vi "Configure Valve.vi"(6 "Three Way Valve Position (0:None)":u16(ring) items=["None", "Bypass", "Input", "Output"], 7 "Valve Type (0:None)":u16(ring) items=["None", "3 Way Non-Distribution", "3 Way Distribution", "4 Way Non-Distribution", "4 Way Distribution", "5 Way Non-Distribution", "5 Way Distribution", "6 Way Non-Distribution", "6 Way Distribution", "8 Way Non-Distribution", "8 Way Distribution", "12 Way Distribution", "2 Way Non-Distribution"], 8 "error in (no error)":errorcluster, 9 "Valve Position (1:Port A)":u16(ring)=1 items=["Port A"=1, "Port B"=2, "Port C"=3, "Port D"=4, "Port E"=5, "Port F"=6, "Port G"=7, "Port H"=8, "Port I"=9, "Port J"=10, "Port K"=11, "Port L"=12], 10 "Address (1)":u16=1 max=15 step=1, 11 "VISA resource name":refnum<visa-resource-name>) -> (0 "error out":errorcluster, 3 "VISA resource name out":refnum<visa-resource-name>)   [LabVIEW 2021, in "Copy of Kloehn V6 Series.lvlib"]
doc: "Configures properties of the valve for the instrument. Things that are customizable include valve type and valve position. It is possible to have more than valve which can be connected via the built in ports or the expansion ports. For those valves that are three way, there are some more options for the positioning of the valve."
uses:
  Copy of Kloehn V6 Series.lvlib
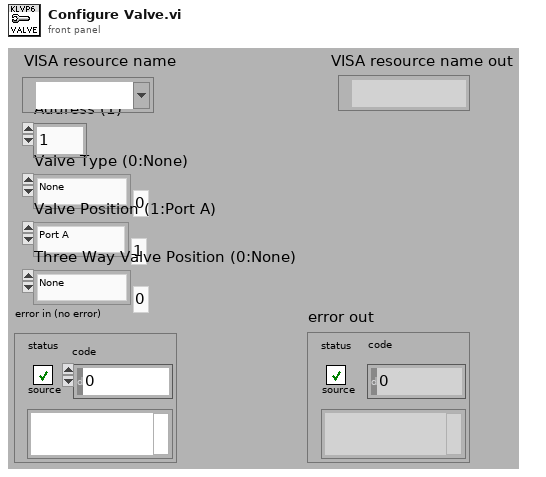
[diagram p1: front panel]
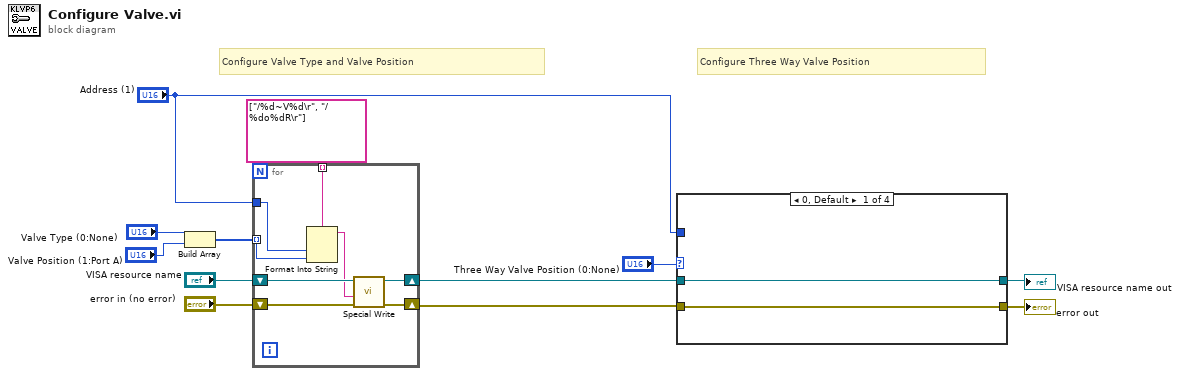
[diagram p0: block diagram]
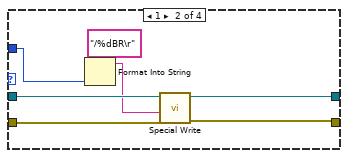
[diagram p2: hidden frame]
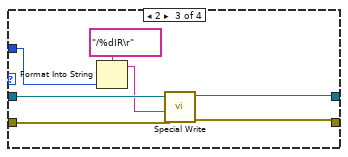
[diagram p3: hidden frame]
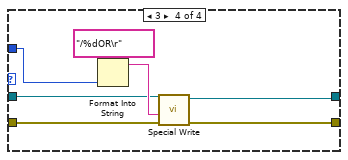
[diagram p4: hidden frame]
diagram:
  # "Configure Three Way Valve Position"
  # "Configure Valve Type and Valve Position"
  n1 = Build Array("Valve Type (0:None)", "Valve Position (1:Port A)") -> (w8:u16[])
  n2 = for {
    tunnel: string[] ["/%d~V%d\r", "/%do%dR\r"] -> [w13] mode=indexing
    tunnel: w8 -> [w20] mode=indexing
    shift-right: [w18] -> w6
    shift-left: "VISA resource name" -> [w17]
    shift-right: [w15] -> w5
    shift-left: "error in (no error)" -> [w14]
    tunnel: "Address (1)" -> [w19]
    n3 = Format Into String(format string=w13, w19, w20) -> (resulting string=w16:string)  [unwired: 2 in, 1 out]
    n4 = call "Special Write.vi"("error in (no error)"=w14, "Send String"=w16, "VISA resource name"=w17) -> ("error out"=w15:errorcluster, "VISA resource name out"=w18:refnum<visa-resource-name>)  [unwired: 4 in, 3 out]
  }
  n5 = case shown="0, Default" "Three Way Valve Position (0:None)" {
    tunnel: [w22 w23 w30 w37] -> w2
    tunnel: w6 -> [w22 w27 w34 w40]
    tunnel: [w21 w24 w31 w38] -> w4
    tunnel: w5 -> [w21 w25 w32 w39]
    tunnel: "Address (1)" -> [_ w29 w35 w42]
    frame 0, Default {
    }
    frame 1 {
      n6 = Format Into String(format string="/%dBR\r" ("Send String"), w29) -> (resulting string=w26:string)  [unwired: 2 in, 1 out]
      n7 = call "Special Write.vi"("error in (no error)"=w25, "Send String"=w26, "VISA resource name"=w27) -> ("error out"=w24:errorcluster, "VISA resource name out"=w23:refnum<visa-resource-name>)  [unwired: 4 in, 3 out]
    }
    frame 2 {
      n8 = Format Into String(format string="/%dIR\r" ("Send String"), w35) -> (resulting string=w33:string)  [unwired: 2 in, 1 out]
      n9 = call "Special Write.vi"("error in (no error)"=w32, "Send String"=w33, "VISA resource name"=w34) -> ("error out"=w31:errorcluster, "VISA resource name out"=w30:refnum<visa-resource-name>)  [unwired: 4 in, 3 out]
    }
    frame 3 {
      n10 = Format Into String(format string="/%dOR\r" ("Send String"), w42) -> (resulting string=w41:string)  [unwired: 2 in, 1 out]
      n11 = call "Special Write.vi"("error in (no error)"=w39, "Send String"=w41, "VISA resource name"=w40) -> ("error out"=w38:errorcluster, "VISA resource name out"=w37:refnum<visa-resource-name>)  [unwired: 4 in, 3 out]
    }
  }
  "error out" <- w4
  "VISA resource name out" <- w2
